vi "MAIN_autofocus_calibration.vi"(0 "Illumination Refnum":refnum<vi>, 1 "Start acquisition":bool, 2 "queue piezo":refnum<queue>, 3 "queue FPGA":refnum<queue>, 5 "Calibration Refnum":refnum<vi>, 9 "Measure QPD":bool caption="Calibration", 11 "error in":errorcluster, 12 "Ref channel":u16(ring) items=["X signal", "Y signal"]) -> (4 "Slope":dbl, 6 "Next task":T1, 10 "Sensitivity (nm)":dbl, 14 "Calibration":cluster{"Y":dbl[], "Y":dbl[]}[](graph), 15 "error out":errorcluster)   [LabVIEW 2015]
uses:
  CONTROLS/Q_MCL_piezo_element.ctl
  CONTROLS/Q_main_element.ctl
  CONTROLS/Q_FPGA_element.ctl
  CONTROLS/Illumination and filters.ctl
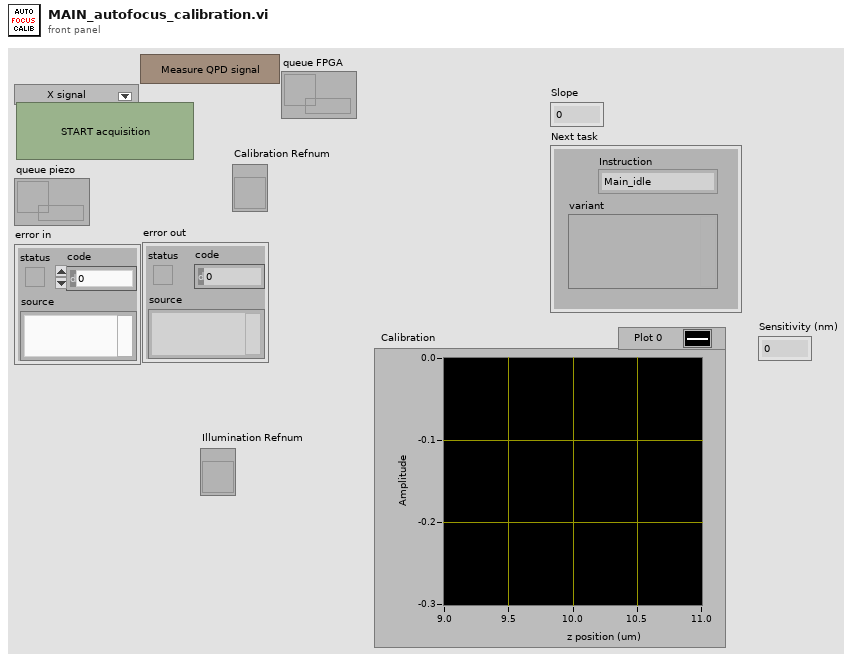
[diagram p1: front panel]
types:
  T1 = typedef "Q_main_element.ctl" = cluster{"variant":variant, "Instruction":enum16{"Main_idle", "Main_initialize", "Main_initialize_TDMS", "Main_initialize_Queue", "Main_error", "Main_DAQ_initialization_results", "Main_ASI_initialization_results", "Main_Piezo_initialization_results", "Main_Valve_initialization_results", "Main_Pump_initialization_results", "Main_CAMERA_initialization_results", "Main_FPGA_initialization_results", "Main_DAQ_error", "Main_ASI_error", "Main_Piezo_error", "Main_CAMERA_error", "Main_Valve_error", "Main_Pump_error", "Main_FPGA_error", "Main_start_acquiring", "Main_not_acquiring", "Main_acquiring", "Main_stop_acquiring", "Main_change_exposure", "Main_change_z_scan_parameters", "Main_define_ROI", "Main_define_mosaic", "Main_read_kinetic_time", "Main_cooler", "Main_read_temperature", "Main_save_XY", "Main_load_XY", "Main_discard_XY", "Main_move_to_XY", "Main_measure_QPD", "Main_autofocus_calibration", "Main_autofocus_initialization", "Main_autofocus_stop", "Main_save_PID", "Main_change_H_valve_position", "Main_two_way_valve", "Main_save_movie", "Main_init_single_scan", "Main_single_scan", "Main_stop_single_scan", "Main_merFISH_illumination_parameters", "Main_merFISH_buffer_probe_list", "Main_merFISH_injections_procedure", "Main_merFISH_save_setpoint", "Main_merFISH_DAPI_parameters", "Main_merFISH_Brightfield_parameters", "Main_merFISH_save_embryo_ROI", "Main_merFISH_init", "Main_merFISH_resume", "Main_merFISH_start_autofocus", "Main_merFISH_open_close_valve_merFISH", "Main_merFISH_open_close_valve_photobleaching", "Main_merFISH_hybridization", "Main_merFISH_move_to_ROI", "Main_merFISH_wait_stabilization", "Main_merFISH_move_to_REF", "Main_merFISH_scan", "Main_merFISH_photobleaching_injection", "Main_merFISH_photobleaching", "Main_merFISH_send_email", "Main_merFISH_close", "Main_STOP"}}
  T2 = typedef "Q_FPGA_element.ctl" = cluster{"variant":variant, "Instruction":enum16{"FPGA_idle", "FPGA_initialize", "FPGA_error", "FPGA_security_stop", "FPGA_laser", "FPGA_start_stop_measure_QPD", "FPGA_measure_QPD", "FPGA_measure_QPD_noise", "FPGA_stop_measure_QPD", "FPGA_init_autofocus", "FPGA_init_single_scan", "FPGA_stop_single_scan", "FPGA_init_merFISH", "FPGA_measure_QPD_merFISH", "FPGA_init_scan_merFISH", "FPGA_scan_merFISH", "FPGA_close_merFISH", "FPGA_stop"}}
  T3 = typedef "Illumination and filters.ctl" = cluster{"BF ":dbl, "641":dbl, "561":dbl, "488":dbl, "405":dbl, "ZERO ALL":bool}
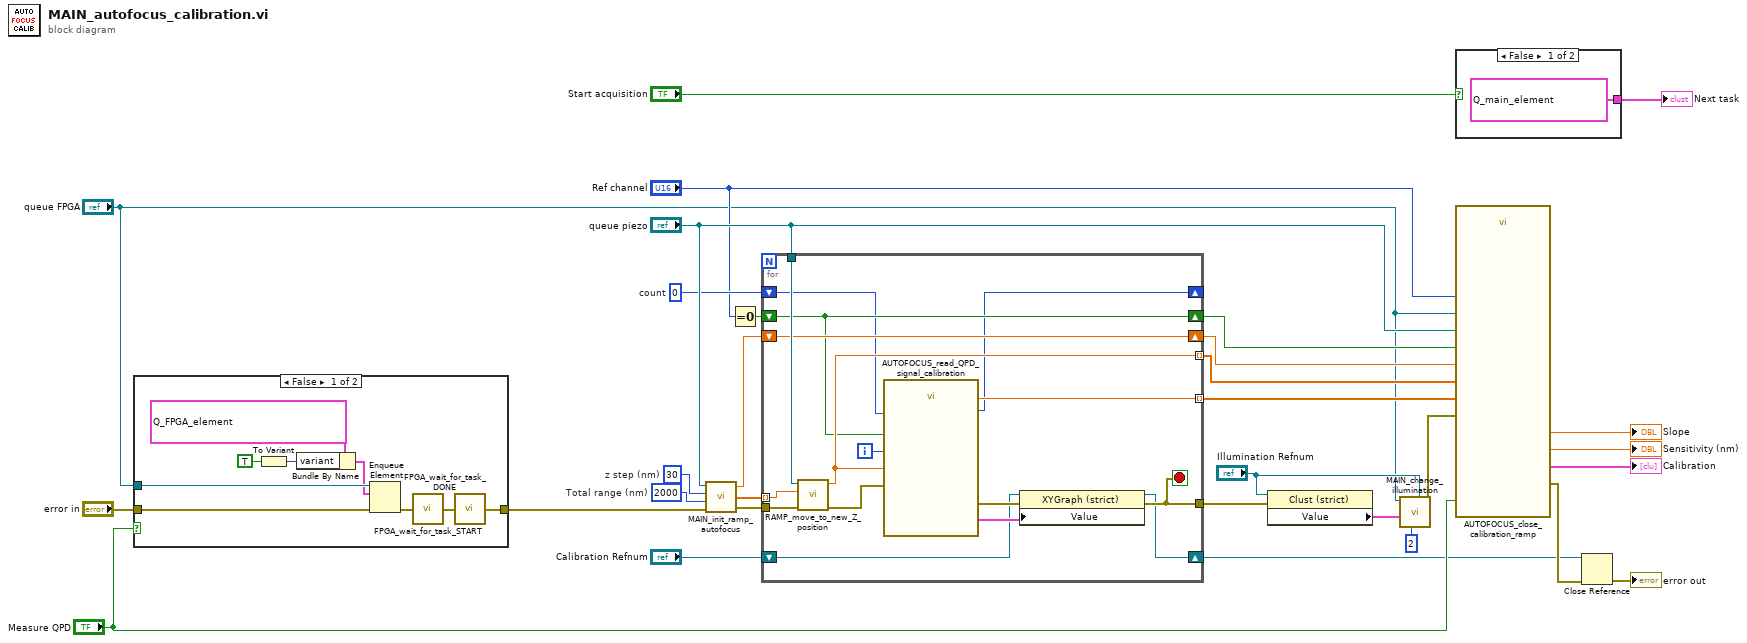
[diagram p0: block diagram]
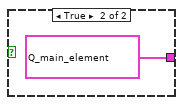
[diagram p3: hidden frame]
diagram:
  w10 = u32 0  # count
  w31 = u32 2000  # Total range (nm)
  w30 = u32 30  # z step (nm)
  n1 = case shown="False" "Measure QPD" {
    tunnel: "error in" -> [w39 w41]
    tunnel: "queue FPGA" -> [w40 _]
    tunnel: [w32 w41] -> w11
    frame False {
      n2 = To Variant(anything=TRUE) -> (Variant=w37:variant)
      n3 = Bundle By Name(cluster=T2 {"variant"=variant, "Instruction"=enum."FPGA_start_stop_measure_QPD"} ("element"), "variant"=w37) -> (w35:T2)
      n4 = Enqueue Element(queue=w40, element=w35, error in (no error)=w39) -> (error out=w34:errorcluster)  [unwired: 1 in, 2 out]
      n5 = call "FPGA_wait_for_task_START.vi"("error in"=w34) -> ("error out"=w33:errorcluster)
      n6 = call "FPGA_wait_for_task_DONE.vi"("error in"=w33) -> ("error out"=w32:errorcluster)
    }
    frame True {
    }
  }
  n7 = call "MAIN_init_ramp_autofocus.vi"("error in"=w11, "Total range (nm)"=w31, "z step (nm)"=w30, "queue piezo"="queue piezo") -> ("error out"=w21:errorcluster, "Ramp"=w22:dbl[], "z0"=w24:dbl)
  n8 = Equal To 0?(x="Ref channel") -> (x = 0?=w23:bool)
  n9 = for {
    tunnel: w21 -> [w57]
    tunnel: w22 -> [w56] mode=indexing
    tunnel: [w46] -> w4
    tunnel: "queue piezo" -> [w55]
    tunnel: [w52] -> w27 mode=indexing
    tunnel: [w51] -> w26 mode=indexing
    shift-right: [w50] -> w28
    shift-left: w24 -> [w50]
    shift-right: [w49] -> w29
    shift-left: w23 -> [w49]
    shift-right: [w45] -> w7
    shift-left: "Calibration Refnum" -> [w44]
    shift-right: [w42] -> _
    shift-left: w10 -> [w43]
    i -> [w53]
    stop <- w46 stop-if-true
    n10 = call "RAMP_move_to_new_Z_position.vi"("error in"=w57, "Z"=w56, "queue piezo"=w55) -> ("error out"=w54:errorcluster, "z"=w52:dbl)  [unwired: 3 in]
    n11 = call "AUTOFOCUS_read_QPD_signal_calibration.vi"("previous count"=w43, "iteration"=w53, "error in"=w54, "z"=w52, "channel"=w49) -> ("error out"=w48:errorcluster, "new count"=w42:u32, "QPD"=w51:dbl, "Calibration"=w47:cluster{"Y":dbl[], "Y":dbl[]}[])  [unwired: 1 in]
    n12 = property class="XYGraph (strict)"(reference=w44, error in=w48, "Value"=w47) -> (reference out=w45:refnum<vi>, error out=w46:errorcluster)
  }
  n13 = property class="Clust (strict)"(reference="Illumination Refnum", error in=w4) -> ("Value"=w2:T3)  [unwired: 2 out]
  n14 = call "MAIN_change_illumination.vi"("Illumination Refnum"="Illumination Refnum", "task number"=2, "Illumination control"=w2, "queue FPGA"="queue FPGA") -> ("error out"=w6:errorcluster)  [unwired: 7 in]
  n15 = case shown="False" "Start acquisition" {
    tunnel: [T1 {"variant"=variant, "Instruction"=enum."Main_not_acquiring"} ("Q_main_element") T1 {"variant"=variant, "Instruction"=enum."Main_acquiring"} ("Q_main_element")] -> w18
    frame False {
    }
    frame True {
    }
  }
  "Next task" <- w18
  n16 = call "AUTOFOCUS_close_calibration_ramp.vi"("queue piezo"="queue piezo", "z0"=w28, "Ref channel"="Ref channel", "queue FPGA"="queue FPGA", "Measure QPD"="Measure QPD", "Channel"=w29, "error in"=w6, "QPD array"=w26, "Z array"=w27) -> ("Calibration"=→"Calibration":cluster{"Y":dbl[], "Y":dbl[]}[], "Slope"=→"Slope":dbl, "Sensitivity (nm)"=→"Sensitivity (nm)":dbl, "error out"=w14:errorcluster)  [unwired: 3 in]
  n17 = Close Reference(reference=w7, error in (no error)=w14) -> (error out=→"error out":errorcluster)
